vi "Hide Subpanel.vi"(8 "error in (no error)":errorcluster, 10 "Subpanel Name":string, 11 "UI Controller in":refnum<class "UI Controller.lvclass">) -> (0 "error out":errorcluster, 3 "UI Controller out":refnum<class "UI Controller.lvclass">)   [LabVIEW 2020, in "UI Controller.lvlib" / "UI Controller.lvclass"]
uses:
  UI Controller.lvclass
  C:/Program Files/National Instruments/LabVIEW 2020/vi.lib/ActorFrameworkMVC/View Controller/View Controller/View Controller.lvclass
  <vilib>/ActorFrameworkMVC/View Controller/View Controller/View Controller.lvclass
panel:
  # "NOTICE -- YOU MUST LEAVE THIS NOTICE IN PLACE.\n\nCopyright (c) 2017, LIANG LIU Shawn.Liu.cn@gmail.com\nAll rights reserved.\n\nRedistribution and use in source and binary forms, with or without modification, are permitted provided that the following conditions are met:\n-Redistributions of source code must retain the above copyright notice, this list of conditions and the following disclaimer.\n-Redistributions in binary form must reproduce the above copyright notice, this list of conditions and the following disclaimer in the documentation and/or other materials provided with the distribution.\n-Neither the name of the eLp nor the names of its contributors may be used to endorse or promote products derived from this software without specific prior written permission.\n\nTHIS SOFTWARE IS PROVIDED BY THE COPYRIGHT HOLDERS AND CONTRIBUTORS \"AS IS\" AND ANY EXPRESS OR IMPLIED WARRANTIES, INCLUDING, BUT NOT LIMITED TO, THE IMPLIED WARRANTIES OF MERCHANTABILITY AND FITNESS FOR A PARTICULAR PURPOSE ARE DISCLAIMED. IN NO EVENT SHALL THE COPYRIGHT HOLDER OR CONTRIBUTORS BE LIABLE FOR ANY DIRECT, INDIRECT, INCIDENTAL, SPECIAL, EXEMPLARY, OR CONSEQUENTIAL DAMAGES (INCLUDING, BUT NOT LIMITED TO, PROCUREMENT OF SUBSTITUTE GOODS OR SERVICES; LOSS OF USE, DATA, OR PROFITS; OR BUSINESS INTERRUPTION) HOWEVER CAUSED AND ON ANY THEORY OF LIABILITY, WHETHER IN CONTRACT, STRICT LIABILITY, OR TORT (INCLUDING NEGLIGENCE OR OTHERWISE) ARISING IN ANY WAY OUT OF THE USE OF THIS SOFTWARE, EVEN IF ADVISED OF THE POSSIBILITY OF SUCH DAMAGE."
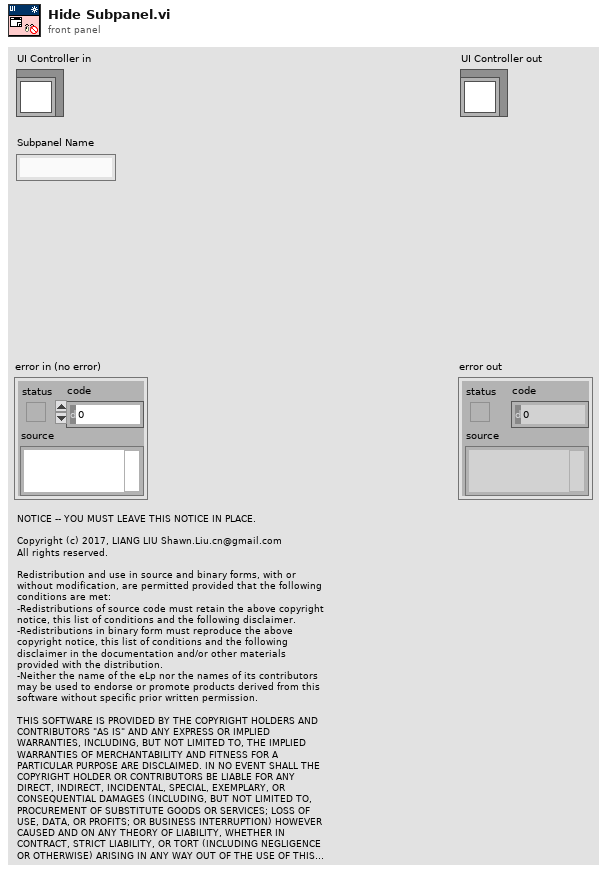
[diagram p1: front panel]
types:
  T1 = typedef "LVBoundsTypeDef.ctl" = cluster{"Width":u32, "Height":u32}
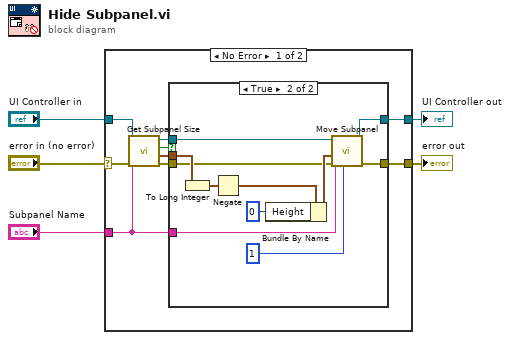
[diagram p0: block diagram]
diagram:
  n1 = case shown="No Error" "error in (no error)" {
    selector: "error in (no error)" -> [w13 w29]
    tunnel: "Subpanel Name" -> [w14 _]
    tunnel: "UI Controller in" -> [w12 w28]
    tunnel: [w11 w29] -> w2
    tunnel: [w10 w28] -> w1
    frame No Error {
      n2 = call <vilib>:"Get Subpanel Size.vi"("error in (no error)"=w13, "Subpanel Name"=w14, "View Controller in"=w12) -> ("error out"=w6:errorcluster, "Subpanel Size"=w7:T1, "Found?"=w8:bool, "View Controller out"=w9:refnum<class "UI Controller.lvclass">)  [unwired: 5 in]
      n3 = case shown="True" w8 {
        tunnel: w9 -> [w15 w27]
        tunnel: w14 -> [_ w26]
        tunnel: w7 -> [_ w25]
        tunnel: w6 -> [w16 w20]
        tunnel: [w16 w19] -> w11
        tunnel: [w15 w18] -> w10
        frame False {
        }
        frame True {
          n4 = To Long Integer(number=w25) -> (32bit integer=w24:cluster{"Width":i32, "Height":i32})
          n5 = Negate(x=w24) -> (-x=w22:cluster{"Width":i32, "Height":i32})
          n6 = Bundle By Name(cluster=w22, "Height"=0) -> (w23:cluster{"Width":i32, "Height":i32})
          n7 = call-dynamic "Move Subpanel.vi"("Loop Number (16)"=1, "error in (no error)"=w20, "Position"=w23, "Subpanel Name"=w26, "View Controller in"=w27) -> ("error out"=w19:errorcluster, "View Controller out"=w18:refnum<class "UI Controller.lvclass">)  [unwired: 5 in]
        }
      }
    }
    frame Error {
    }
  }
  "error out" <- w2
  "UI Controller out" <- w1
